vi "drawsquare.vi"() -> ()   [LabVIEW 2025]
uses:
  <vilib>/picture/picture.llb/Draw True-Color Pixmap.vi
panel:
  out "col":dbl
  out "row":dbl
  in  "pen 2":T1={"Width"=1, "Style"=enum."Solid"}
  out "map data":dbl[][](array[numeric])
  in  "pen":T1={"Width"=1, "Style"=enum."Solid"}
  in  "stop":bool
  in  "grid size":dbl
  out "2D Picture":picture
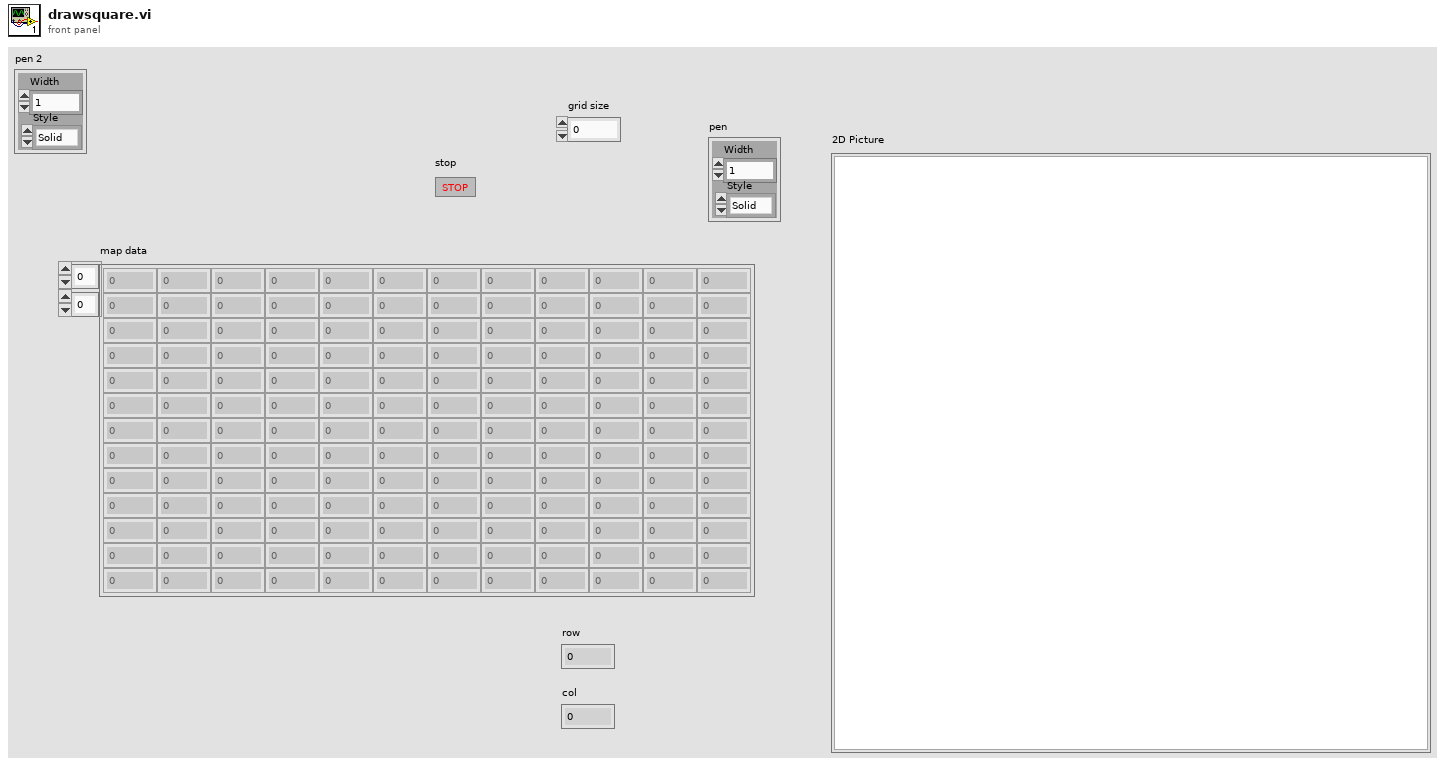
[diagram p1: front panel]
types:
  T1 = cluster{"Width":i16, "Style":enum32{"Solid", "Dash", "Dot", "DashDot", "DashDotDot"}}
  T2 = typedef "imagedata.ctl" = cluster{"image type":i32, "image depth":i32, "image":u8[], "mask":u8[], "colors":u32[], "Rectangle":cluster{"left":i16, "top":i16, "right":i16, "bottom":i16}}
  T3 = typedef "LVPoint32TypeDef.ctl" = cluster{"Horizontal":i32, "Vertical":i32}
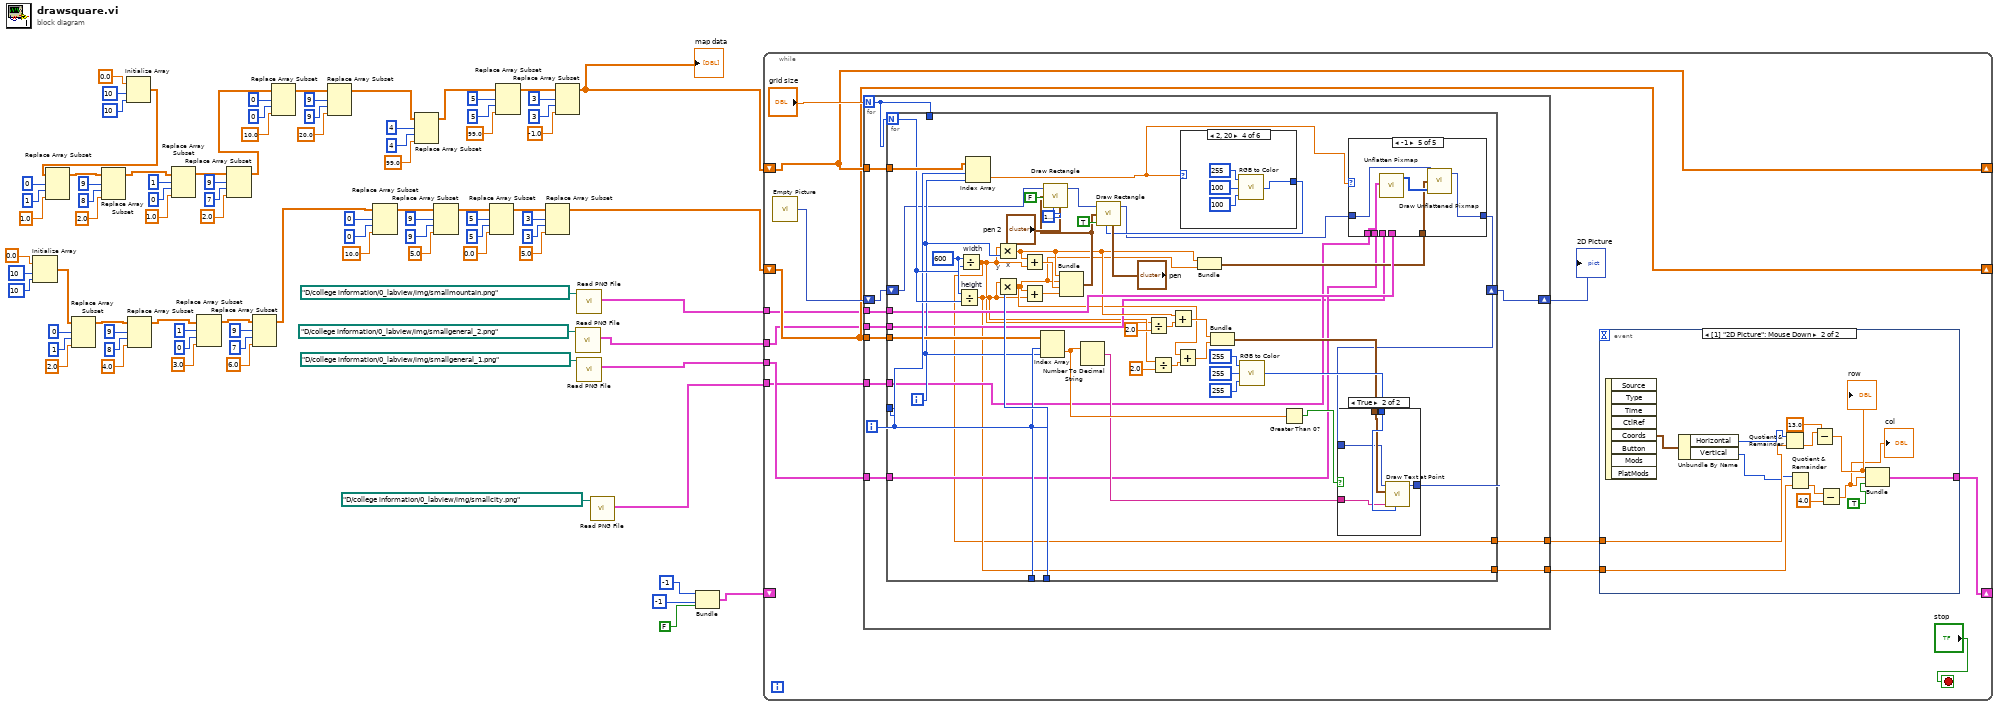
[diagram p0: block diagram]
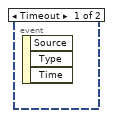
[diagram p2: hidden frame]
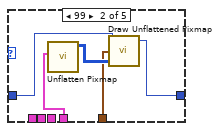
[diagram p4: hidden frame]
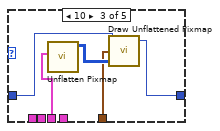
[diagram p5: hidden frame]
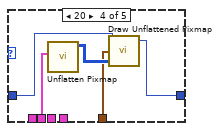
[diagram p6: hidden frame]
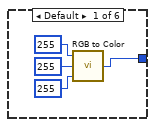
[diagram p8: hidden frame]
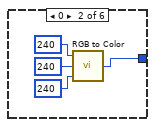
[diagram p9: hidden frame]
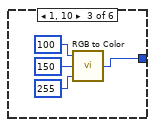
[diagram p10: hidden frame]
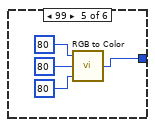
[diagram p11: hidden frame]
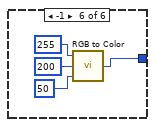
[diagram p12: hidden frame]
diagram:
  n1 = Initialize Array(0.0, 10, 10) -> (w11:dbl[][])
  n2 = Replace Array Subset(array=w11, new element=2.0 ("new element/subarray"), index (row)=0, index (col)=1 ("index (row)")) -> (w10:dbl[][])
  n3 = Initialize Array(0.0, 10, 10) -> (w26:dbl[][])
  n4 = Replace Array Subset(array=w26, new element=1.0 ("new element/subarray"), index (row)=0, index (col)=1 ("index (row)")) -> (w25:dbl[][])
  n5 = Replace Array Subset(array=w25, new element=2.0 ("new element/subarray"), index (row)=9, index (col)=8 ("index (row)")) -> (w24:dbl[][])
  n6 = Replace Array Subset(array=w10, new element=4.0 ("new element/subarray"), index (row)=9, index (col)=8 ("index (row)")) -> (w9:dbl[][])
  n7 = Replace Array Subset(array=w24, new element=1.0 ("new element/subarray"), index (row)=1, index (col)=0 ("index (row)")) -> (w40:dbl[][])
  n8 = Replace Array Subset(array=w9, new element=3.0 ("new element/subarray"), index (row)=1, index (col)=0 ("index (row)")) -> (w8:dbl[][])
  n9 = Replace Array Subset(array=w40, new element=2.0 ("new element/subarray"), index (row)=9, index (col)=7 ("index (row)")) -> (w33:dbl[][])
  n10 = Replace Array Subset(array=w8, new element=6.0 ("new element/subarray"), index (row)=9, index (col)=7 ("index (row)")) -> (w7:dbl[][])
  n11 = Replace Array Subset(array=w33, new element=10.0 ("new element/subarray"), index (row)=0, index (col)=0 ("index (row)")) -> (w73:dbl[][])
  n12 = Replace Array Subset(array=w73, new element=20.0 ("new element/subarray"), index (row)=9, index (col)=9 ("index (row)")) -> (w46:dbl[][])
  n13 = Replace Array Subset(array=w7, new element=10.0 ("new element/subarray"), index (row)=0, index (col)=0 ("index (row)")) -> (w68:dbl[][])
  n14 = Replace Array Subset(array=w46, new element=99.0 ("new element/subarray"), index (row)=4, index (col)=4 ("index (row)")) -> (w45:dbl[][])
  n15 = Replace Array Subset(array=w68, new element=5.0 ("new element/subarray"), index (row)=9, index (col)=9 ("index (row)")) -> (w69:dbl[][])
  n16 = Replace Array Subset(array=w69, new element=0.0 ("new element/subarray"), index (row)=5, index (col)=5 ("index (row)")) -> (w70:dbl[][])
  n17 = Replace Array Subset(array=w45, new element=99.0 ("new element/subarray"), index (row)=5, index (col)=5 ("index (row)")) -> (w72:dbl[][])
  n18 = Replace Array Subset(array=w70, new element=5.0 ("new element/subarray"), index (row)=3, index (col)=3 ("index (row)")) -> (w52:dbl[][])
  n19 = Replace Array Subset(array=w72, new element=-1.0 ("new element/subarray"), index (row)=3, index (col)=3 ("index (row)")) -> (w71:dbl[][])
  "map data" <- w71
  n20 = call <vilib>:"Read PNG File.vi"("path to PNG file"=path "D:/college information/0_labview/img/smallgeneral_2.png") -> ("image data"=w5:T2)  [unwired: 8 in, 2 out]
  n21 = call <vilib>:"Read PNG File.vi"("path to PNG file"=path "D:/college information/0_labview/img/smallmountain.png") -> ("image data"=w50:T2)  [unwired: 8 in, 2 out]
  n22 = call <vilib>:"Read PNG File.vi"("path to PNG file"=path "D:/college information/0_labview/img/smallgeneral_1.png") -> ("image data"=w42:T2)  [unwired: 8 in, 2 out]
  n23 = call <vilib>:"Read PNG File.vi"("path to PNG file"=path "D:/college information/0_labview/img/smallcity.png") -> ("image data"=w41:T2)  [unwired: 8 in, 2 out]
  n24 = Bundle(-1, -1, FALSE) -> (w1:cluster{i32, i32, bool})  [unwired: 1 in]
  n25 = while {
    shift-right: [w97] -> _
    shift-left: w71 -> [w97]
    shift-right: [w96] -> _
    shift-left: w52 -> [w96]
    tunnel: w50 -> [w95]
    tunnel: w42 -> [w94]
    tunnel: w41 -> [w93]
    tunnel: w5 -> [w92]
    shift-right: [w89] -> _
    shift-left: w1 -> [_]
    stop <- "stop" stop-if-true
    n26 = call "Empty Picture"() -> ("empty picture"=w98:picture)
    n27 = for {
      N: "grid size" -> [w124]
      shift-right: [w121] -> w99
      shift-left: w98 -> [w126]
      tunnel: w97 -> [w125]
      tunnel: w96 -> [w123]
      tunnel: w95 -> [w120]
      tunnel: w94 -> [w119]
      tunnel: w93 -> [w118]
      tunnel: w92 -> [w117]
      tunnel: [w116] -> w91
      tunnel: [w115] -> w90
      i -> [w122]
      n28 = for {
        N: w124 -> [w166]
        tunnel: w122 -> [w171]
        shift-right: [w146] -> w121
        shift-left: w126 -> [w144]
        tunnel: w125 -> [w167]
        tunnel: w124 -> [_]
        tunnel: w122 -> [w165]
        tunnel: w123 -> [w163]
        tunnel: w122 -> [w162]
        tunnel: w120 -> [w137]
        tunnel: w119 -> [w131]
        tunnel: w118 -> [w130]
        tunnel: w117 -> [w129]
        tunnel: [w128] -> w116
        tunnel: [w127] -> w115
        i -> [w161]
        w172 = 600
        n29 = Divide "height"(x=w172, y=w166) -> (x/y=w128:dbl)
        n30 = Divide "width"(x=w172, y=w166) -> (x/y=w127:dbl)
        n31 = Index Array(array=w167, index (row)=w165, index (col)=w161) -> (element=w132:dbl)
        n32 = Multiply "x"(x=w127, y=w161) -> (x*y=w135:dbl)
        n33 = Multiply "y"(x=w128, y=w171) -> (x*y=w134:dbl)
        n34 = Add(x=w135, y=w127) -> (x+y=w170:dbl)
        n35 = Add(x=w134, y=w128) -> (x+y=w169:dbl)
        n36 = Index Array(array=w163, index (row)=w162, index (col)=w161) -> (element=w150:dbl)
        n37 = Bundle(w135, w134, w170, w169) -> (w136:cluster{dbl, dbl, dbl, dbl})  [unwired: 1 in]
        n38 = call <vilib>:"Draw Rectangle.vi"("picture"=w144, "rect"=w136, "fill?(F)"=FALSE, "color(black)"=u32 16777222, "pen"="pen 2") -> ("new picture"=w143:picture)  [unwired: 4 in]
        n39 = Number To Decimal String(number=w150) -> (decimal integer string=w148:string)  [unwired: 1 in]
        n40 = Divide(x=w127, y=2.0) -> (x/y=w159:dbl)
        n41 = Divide(x=w128, y=2.0) -> (x/y=w158:dbl)
        n42 = Add(x=w135, y=w159) -> (x+y=w156:dbl)
        n43 = Add(x=w134, y=w158) -> (x+y=w155:dbl)
        n44 = case shown="2, 20" w132 {
          tunnel: [w200 w204 w208 w212 w216 w220] -> w164
          frame Default {
            n45 = call <vilib>:"RGB to Color.vi"("B"=255, "G"=255, "R"=255) -> ("Color"=w200:u32)
          }
          frame 0 {
            n46 = call <vilib>:"RGB to Color.vi"("B"=240, "G"=240, "R"=240) -> ("Color"=w204:u32)
          }
          frame 1, 10 {
            n47 = call <vilib>:"RGB to Color.vi"("B"=255, "G"=150, "R"=100) -> ("Color"=w208:u32)
          }
          frame 2, 20 {
            n48 = call <vilib>:"RGB to Color.vi"("B"=100, "G"=100, "R"=255) -> ("Color"=w212:u32)
          }
          frame 99 {
            n49 = call <vilib>:"RGB to Color.vi"("B"=80, "G"=80, "R"=80) -> ("Color"=w216:u32)
          }
          frame -1 {
            n50 = call <vilib>:"RGB to Color.vi"("B"=50, "G"=200, "R"=255) -> ("Color"=w220:u32)
          }
        }
        n51 = call <vilib>:"Draw Rectangle.vi"("picture"=w143, "rect"=w136, "fill?(F)"=TRUE, "color(black)"=w164, "pen"="pen") -> ("new picture"=w139:picture)  [unwired: 4 in]
        n52 = Bundle(w135, w134) -> (w133:cluster{dbl, dbl})  [unwired: 1 in]
        n53 = Bundle(w156, w155) -> (w147:cluster{dbl, dbl})  [unwired: 1 in]
        n54 = call <vilib>:"RGB to Color.vi"("B"=255, "G"=255, "R"=255) -> ("Color"=w149:u32)
        n55 = Greater Than 0?(x=w150) -> (x > 0?=w151:bool)
        n56 = case shown="-1" w132 {
          tunnel: w139 -> [w173 w176 w182 w187 w192]
          tunnel: [w173 w174 w180 w185 w190] -> w138
          tunnel: w137 -> [_ w177 _ _ _]
          tunnel: w133 -> [_ w175 w181 w186 w191]
          tunnel: w131 -> [_ _ _ w184 _]
          tunnel: w130 -> [_ _ _ _ w189]
          tunnel: w129 -> [_ _ w179 _ _]
          frame 0, Default {
          }
          frame 99 {
            n57 = call <vilib>:"Unflatten Pixmap.vi"("image data"=w177) -> ("24-bit pixmap"=w178:u32[][])  [unwired: 4 in, 6 out]
            n58 = call-poly <vilib>:"Draw Unflattened Pixmap.vi"("picture"=w176, "top left point(0, 0)"=w175, "data (RGB format)"=w178) -> ("new picture"=w174:picture)  [unwired: 6 in]
          }
          frame 10 {
            n59 = call <vilib>:"Unflatten Pixmap.vi"("image data"=w179) -> ("24-bit pixmap"=w183:u32[][])  [unwired: 4 in, 6 out]
            n60 = call-poly <vilib>:"Draw Unflattened Pixmap.vi"("picture"=w182, "top left point(0, 0)"=w181, "data (RGB format)"=w183) -> ("new picture"=w180:picture)  [unwired: 6 in]
          }
          frame 20 {
            n61 = call <vilib>:"Unflatten Pixmap.vi"("image data"=w184) -> ("24-bit pixmap"=w188:u32[][])  [unwired: 4 in, 6 out]
            n62 = call-poly <vilib>:"Draw Unflattened Pixmap.vi"("picture"=w187, "top left point(0, 0)"=w186, "data (RGB format)"=w188) -> ("new picture"=w185:picture)  [unwired: 6 in]
          }
          frame -1 {
            n63 = call <vilib>:"Unflatten Pixmap.vi"("image data"=w189) -> ("24-bit pixmap"=w193:u32[][])  [unwired: 4 in, 6 out]
            n64 = call-poly <vilib>:"Draw Unflattened Pixmap.vi"("picture"=w192, "top left point(0, 0)"=w191, "data (RGB format)"=w193) -> ("new picture"=w190:picture)  [unwired: 6 in]
          }
        }
        n65 = case shown="True" w151 {
          tunnel: w149 -> [_ w199]
          tunnel: w148 -> [_ w198]
          tunnel: w147 -> [_ w197]
          tunnel: w138 -> [w194 w196]
          tunnel: [w194 w195] -> w146
          frame False {
          }
          frame True {
            n66 = call <vilib>:"Draw Text at Point.vi"("text color(black)"=w199, "text"=w198, "origin"=w197, "picture"=w196) -> ("new picture"=w195:picture)  [unwired: 6 in, 1 out]
          }
        }
      }
    }
    "2D Picture" <- w99
    n67 = event shown="[1] \"2D Picture\": Mouse Down" {
      selector: _ -> [_ _]
      dyn-events: _ -> [_ _]
      timeout: _ -> [_ _]
      tunnel: w91 -> [_ w112]
      tunnel: w90 -> [_ w113]
      tunnel: [_ w110] -> w89
      event Timeout {
        n68 = event-data() -> ()  [unwired: 1 in, 3 out]
      }
      event "2D Picture": Mouse Down {
        n69 = event-data() -> ("Coords"=w114:T3)  [unwired: 1 in, 7 out]
        n70 = Unbundle By Name(w114) -> ("Horizontal"=w109:i32, "Vertical"=w108:i32)
        n71 = Quotient & Remainder(x=w109, y=w113) -> (floor(x/y)=w106:dbl)  [unwired: 1 out]
        n72 = Quotient & Remainder(x=w108, y=w112) -> (floor(x/y)=w104:dbl)  [unwired: 1 out]
        n73 = Subtract(x=w106, y=13.0) -> (x-y=w107:dbl)
        "row" <- w107
        n74 = Subtract(x=w104, y=4.0) -> (x-y=w103:dbl)
        "col" <- w103
        n75 = Bundle(w107, w103, TRUE) -> (w110:cluster{dbl, dbl, bool})  [unwired: 1 in]
      }
    }
  }
